vi "tag bus to parameters.vi"(9 "indices":T1, 11 "tag bus in":T3) -> (2 "data cluster":T2, 3 "tag bus out":T3)   [LabVIEW 2017, in "Convert Bool to Velocity runtime.lvclass"]
uses:
  Convert Bool to Velocity runtime.lvclass
  <vilib>/NI/Tag Bus/table/data table.ctl
  parameter user data.ctl
  configuration/parameter data indices.ctl
  <vilib>/NI/Tag Bus/table/data polymorphs/read one/read Boolean.vi
  <vilib>/NI/Tag Bus/table/data table.lvlib
  configuration/Convert Bool to Velocity configuration.lvclass
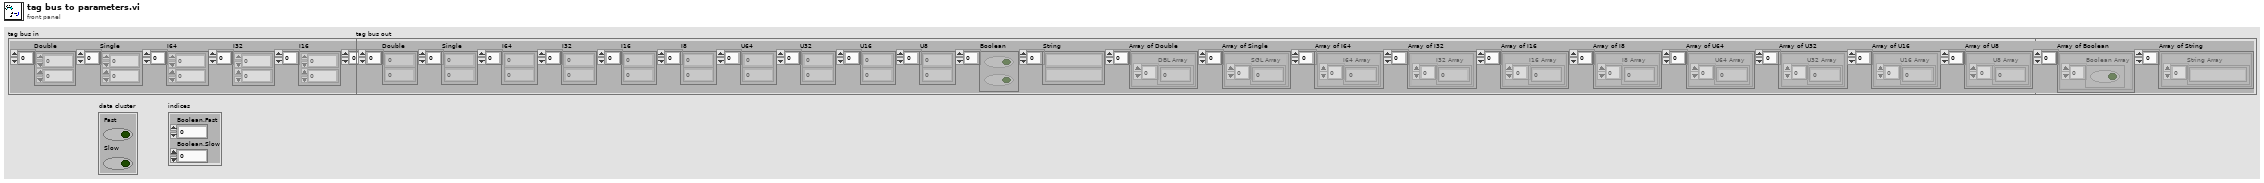
[diagram p1: front panel]
types:
  T1 = typedef "Convert Bool to Velocity configuration.lvclass/parameter data indices.ctl" = cluster{"Boolean.Fast":i32, "Boolean.Slow":i32}
  T2 = typedef "Convert Bool to Velocity runtime.lvclass/parameter user data.ctl" = cluster{"Fast":bool, "Slow":bool}
  T3 = typedef "tag bus.lvlib/data table.lvlib/data table.ctl" = cluster{"Double":dbl[], "Single":sgl[], "I64":i64[], "I32":i32[], "I16":i16[], "I8":i8[], "U64":u64[], "U32":u32[], "U16":u16[], "U8":u8[], "Boolean":bool[], "String":string[], "Array of Double":cluster{"DBL Array":dbl[]}[], "Array of Single":cluster{"SGL Array":sgl[]}[], "Array of I64":cluster{"I64 Array":i64[]}[], "Array of I32":cluster{"I32 Array":i32[]}[], "Array of I16":cluster{"I16 Array":i16[]}[], "Array of I8":cluster{"I8 Array":i8[]}[], "Array of U64":cluster{"U64 Array":u64[]}[], "Array of U32":cluster{"U32 Array":u32[]}[], "Array of U16":cluster{"U16 Array":u16[]}[], "Array of U8":cluster{"U8 Array":u8[]}[], "Array of Boolean":cluster{"Boolean Array":bool[]}[], "Array of String":cluster{"String Array":string[]}[]}
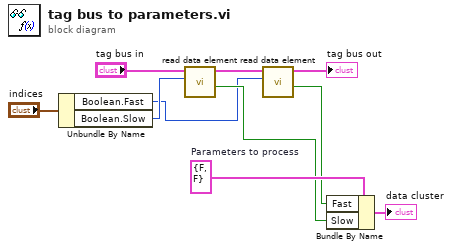
[diagram p0: block diagram]
diagram:
  w9 = T2 {"Fast"=FALSE, "Slow"=FALSE}  # Parameters to process
  n1 = Unbundle By Name("indices") -> ("Boolean.Fast"=w2:i32, "Boolean.Slow"=w5:i32)
  n2 = call-poly <vilib>:"read data element.vi"("index"=w5, "data table in"="tag bus in") -> ("value"=w6:bool, "data table out"=w4:T3)  [unwired: 8 in]
  n3 = call-poly <vilib>:"read data element.vi"("index"=w2, "data table in"=w4) -> ("value"=w3:bool, "data table out"=→"tag bus out":T3)  [unwired: 8 in]
  n4 = Bundle By Name(cluster=w9, "Fast"=w3, "Slow"=w6) -> (→"data cluster":T2)
